vi "String to Version.vi"(0 "Version String":string) -> (2 "Is Pre-Release":bool, 4 "Version":T1, 5 "Pre-Release":string)   [LabVIEW 2020, in "Builder Core.lvlib"]
uses:
  Builder Core.lvlib
  Version.ctl
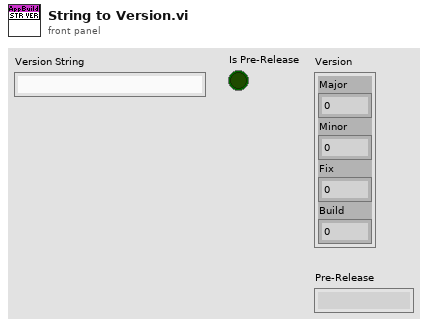
[diagram p1: front panel]
types:
  T1 = typedef "Builder Core.lvlib/Version.ctl" = cluster{"Major":u16, "Minor":u16, "Fix":u16, "Build":u16}
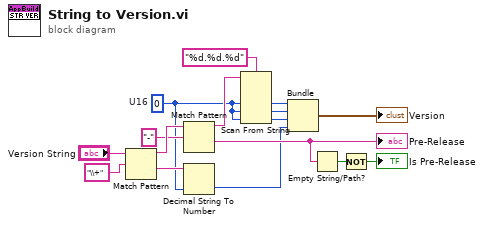
[diagram p0: block diagram]
diagram:
  w6 = u16 0  # U16
  n1 = Match Pattern(string="Version String", regular expression="\\+") -> (before substring=w13:string, after substring=w14:string)  [unwired: 1 in, 2 out]
  n2 = Match Pattern(string=w13, regular expression="-") -> (before substring=w8:string, after substring=w11:string)  [unwired: 1 in, 2 out]
  "Pre-Release" <- w11
  n3 = Decimal String To Number(string=w14, default (0L)=w6) -> (number=w2:u16)  [unwired: 1 in, 1 out]
  n4 = Scan From String(format string="%d.%d.%d", input string=w8, default 1=w6, default 2=w6, default 3=w6) -> (output 1=w5:u16, output 2=w4:u16, output 3=w3:u16)  [unwired: 2 in, 3 out]
  n5 = Bundle("U16"=w5, "U16"=w4, "U16"=w3, w2) -> (→"Version":cluster{"U16":u16, "U16":u16, "U16":u16, u16})  [unwired: 1 in]
  n6 = Empty String/Path?(string/path=w11) -> (empty?=w10:bool)
  n7 = Not(x=w10) -> (.not. x?=→"Is Pre-Release":bool)
